vi "HW Cluster to Classes.vi"(8 "error in (no error)":errorcluster, 11 "real hardware controls":T1 {"color pane" items=["Blue", "Red", "Green", "Saturation", "Value", "Intensity", "Luminance", "Hue", ""]}) -> (0 "error out":errorcluster, 1 "DAQmx Switch out":refnum<class "DAQmx Switch.lvclass">, 2 "DAQmx Servo out":refnum<class "DAQmx Servo.lvclass">, 3 "DAQmx Force Sensor out":refnum<class "DAQmx Force Sensor.lvclass">, 5 "USB Camera out":refnum<class "USB Camera.lvclass">)   [LabVIEW 2020]
uses:
  Sensors/Force Sensors/DAQmx Force Sensor/DAQmx Force Sensor.lvclass
  C:/Users/jharw/Documents/1 Folder to Rule them All/UMD/Inflation-Apparatus/src/Hardware/General Hardware.lvclass
  Inflation Test/Controls/Hardware Options.ctl
  <vilib>/userdefined/High Color/IMAQdx.ctl
  Sensors/Cameras/USB Camera/USB Camera.lvclass
  C:/Users/jharw/Documents/1 Folder to Rule them All/UMD/Inflation-Apparatus/src/Hardware/Sensors/Cameras/Camera.lvclass
  Actuators/Servos/DAQmx Servo/DAQmx Servo.lvclass
  Actuators/Switches/DAQmx Switch/DAQmx Switch.lvclass
  General Hardware.lvclass/General Hardware.ctl
  Sensors/Force Sensors/DAQmx Force Sensor/DAQmx Force Sensor.lvclass/DAQmx Force Sensor.ctl
  Sensors/Cameras/Camera.lvclass/Camera.ctl
  Sensors/Cameras/USB Camera/USB Camera.lvclass/USB Camera.ctl
  Actuators/Servos/DAQmx Servo/DAQmx Servo.lvclass/DAQmx Servo.ctl
  Actuators/Switches/DAQmx Switch/DAQmx Switch.lvclass/DAQmx Switch.ctl
  General Hardware.lvclass
  Sensors/Cameras/Camera.lvclass
panel:
  # "FORCE SENSOR CHANNEL"
  # "SERVO CHANNEL"
  # "LED CHANNEL"
  # "CAMERA PORT"
  # "CAMERA FREQUENCY (HZ):"
  # "FS FREQUENCY (HZ):"
  # "SERVO FREQUENCY (HZ):"
  # "COLOR PANE:"
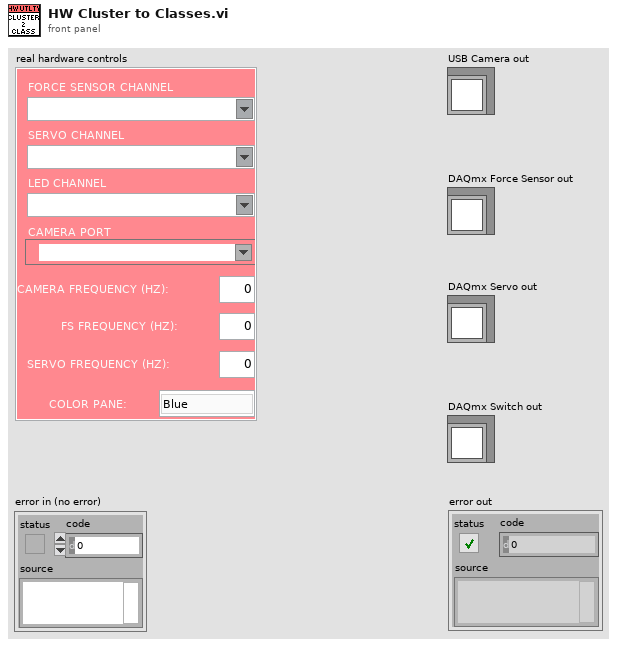
[diagram p1: front panel]
types:
  T1 = typedef "Hardware Options.ctl" = cluster{"fs chan":tag, "servo chan":tag, "led chan":tag, "camera port":T2, "cam freq":dbl, "fs freq":dbl, "color pane":i32, "servo freq":dbl}
  T2 = typedef "IMAQdx.ctl" = refnum<k21>
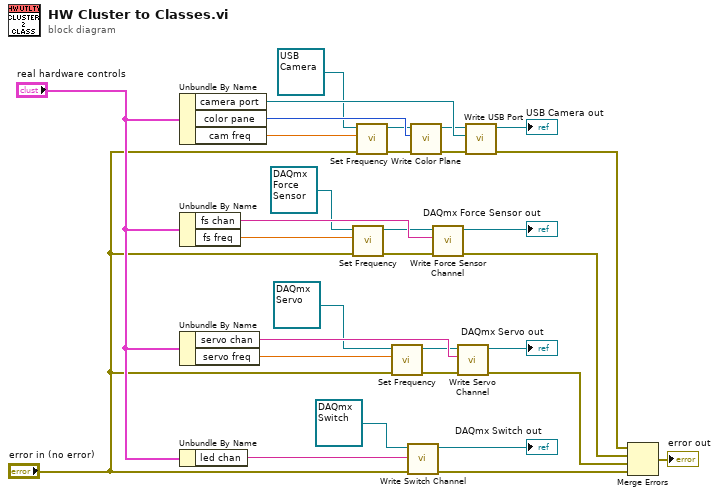
[diagram p0: block diagram]
diagram:
  n1 = Unbundle By Name("real hardware controls") -> ("camera port"=w24:T2, "color pane"=w23:i32, "cam freq"=w19:dbl)
  n2 = Unbundle By Name("real hardware controls") -> ("fs chan"=w31:tag, "fs freq"=w30:dbl)
  n3 = Unbundle By Name("real hardware controls") -> ("servo chan"=w18:tag, "servo freq"=w15:dbl)
  n4 = Unbundle By Name("real hardware controls") -> ("led chan"=w12:tag)
  n5 = call "Set Frequency.vi"("error in (no error)"="error in (no error)", "frequency (Hz)"=w30, "General Hardware in"=refnum<class "DAQmx Force Sensor.lvclass"> refnum ("DAQmx Force Sensor.lvclass")) -> ("error out"=w8:errorcluster, "General Hardware out"=w28:refnum<class "DAQmx Force Sensor.lvclass">)  [unwired: 7 in]
  n6 = call "Set Frequency.vi"("error in (no error)"="error in (no error)", "frequency (Hz)"=w19, "General Hardware in"=refnum<class "USB Camera.lvclass"> refnum ("USB Camera.lvclass")) -> ("error out"=w10:errorcluster, "General Hardware out"=w21:refnum<class "USB Camera.lvclass">)  [unwired: 7 in]
  n7 = call "Set Frequency.vi"("error in (no error)"="error in (no error)", "frequency (Hz)"=w15, "General Hardware in"=refnum<class "DAQmx Servo.lvclass"> refnum ("DAQmx Servo.lvclass")) -> ("error out"=w1:errorcluster, "General Hardware out"=w17:refnum<class "DAQmx Servo.lvclass">)  [unwired: 7 in]
  n8 = call "Write Switch Channel.vi"("error in (no error)"="error in (no error)", "switch phys chan"=w12, "DAQmx Switch in"=refnum<class "DAQmx Switch.lvclass"> refnum ("DAQmx Switch.lvclass")) -> ("error out"=w6:errorcluster, "DAQmx Switch out"=→"DAQmx Switch out":refnum<class "DAQmx Switch.lvclass">)  [unwired: 7 in]
  n9 = call "Write Color Plane.vi"("error in (no error)"=w10, "Color Plane"=w23, "Camera in"=w21) -> ("error out"=w9:errorcluster, "Camera out"=w22:refnum<class "USB Camera.lvclass">)  [unwired: 7 in]
  n10 = call "Write Force Sensor Channel.vi"("error in (no error)"=w8, "fs phys chan"=w31, "DAQmx Force Sensor in"=w28) -> ("error out"=w4:errorcluster, "DAQmx Force Sensor out"=→"DAQmx Force Sensor out":refnum<class "DAQmx Force Sensor.lvclass">)  [unwired: 7 in]
  n11 = call "Write Servo Channel.vi"("error in (no error)"=w1, "servo phys chan"=w18, "DAQmx Servo in"=w17) -> ("error out"=w5:errorcluster, "DAQmx Servo out"=→"DAQmx Servo out":refnum<class "DAQmx Servo.lvclass">)  [unwired: 7 in]
  n12 = call "Write USB Port.vi"("error in (no error)"=w9, "camera session"=w24, "USB Camera in"=w22) -> ("error out"=w3:errorcluster, "USB Camera out"=→"USB Camera out":refnum<class "USB Camera.lvclass">)  [unwired: 7 in]
  n13 = Merge Errors(w3, w4, w5, w6) -> (→"error out":errorcluster)
